vi "Stop Core.vi"(10 "final error code":i32, 11 "PW3390 in":refnum<class "PW3390.lvclass">) -> (3 "PW3390 out":refnum<class "PW3390.lvclass">)   [LabVIEW 2024, in "PW3390 Actor.lvlib" / "PW3390.lvclass"]
doc: "<p>(<strong>Filename</strong>: <span class=\"dnl\">Actor Framework.lvlib:Actor.lvclass:Stop Core.vi</span>)</p>\n<p>Defines what the actor does before it stops. Use the <strong>final error code</strong> input to determine whether the actor shut down in response to an error.</p>\n<p>By default, this method passes the Stop message along to all <a href=\"nihelplauncher://docs/csh?context=lvcore_lvcomm_af_launch_nested_actor\">auto-stop nested actors</a>. A descendant class may override this method to define additional behavior, such as shutting down any processes the actor initiated in its override of the <a href=\"nihelplauncher://docs/csh?context=lvcore_lvcomm_af_actor_core\">Actor Core</a> method.</p>"
uses:
  PW3390.lvclass
  PW3390.lvclass/PW3390.ctl
  <vilib>/ActorFramework/Actor/Actor.lvclass
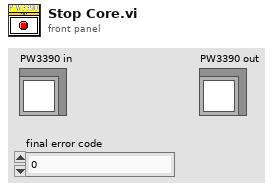
[diagram p1: front panel]
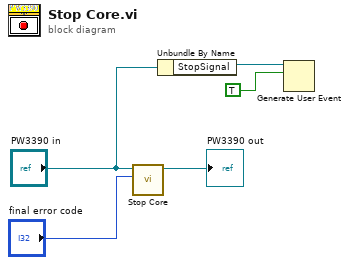
[diagram p0: block diagram]
diagram:
  n1 = call-parent "Stop Core.vi"("final error code"="final error code", "Actor in"="PW3390 in") -> ("Actor out"=→"PW3390 out":refnum<class "PW3390.lvclass">)  [unwired: 9 in]
  n2 = Unbundle By Name("PW3390 in") -> ("StopSignal"=w2:refnum<user-event>)
  n3 = Generate User Event(user event=w2, event data cluster=TRUE) -> ()  [unwired: 2 in, 2 out]
